vi "FT_Get_Event_Status.vi"(0 "Handle":u32) -> (1 "FT_Status":u32(ring) items=["FT_OK", "FT_INVALID_HANDLE", "FT_DEVICE_NOT_FOUND", "FT_DEVICE_NOT_OPENED", "FT_IO_ERROR", "FT_INSUFFICIENT_RESOURCES", "FT_INVALID_PARAMETER", "FT_INVALID_BAUD_RATE", "FT_DEVICE_NOT_OPENED_FOR_ERASE", "FT_DEVICE_NOT_OPENED_FOR_WRITE", "FT_FAILED_TO_WRITE_DEVICE", "FT_EEPROM_READ_FAILED", "FT_EEPROM_WRITE_FAILED", "FT_EEPROM_ERASE_FAILED", "FT_EEPROM_NOT_PRESENT", "FT_EEPROM_NOT_PROGRAMMED", "FT_INVALID_ARGS", "FT_NOT_SUPPORTED", "FT_OTHER_ERROR"], 2 "EventStatus":u32)   [LabVIEW 2019, in "D2XX.lvlib"]
uses:
  D2XX.lvlib
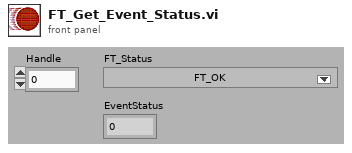
[diagram p1: front panel]
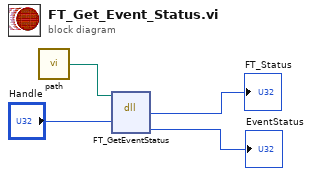
[diagram p0: block diagram]
diagram:
  n1 = call "path.vi"() -> ("lib path"=w1:path)
  n2 = dll-call lib="FTD2XX.dll" fn="FT_GetEventStatus"(path in=w1, "Handle"="Handle") -> (→"FT_Status":u32, "EventStatus"=→"EventStatus":u32)  [unwired: 4 in, 2 out]
